vi "SPI Master.vi"(2 "Data In U32":u32, 3 "Data In U64":u64, 4 "Mode":bool) -> (0 "Data In Out U32":u32, 1 "Data In Out U64":u64)   [LabVIEW 2018]
uses:
  <vilib>/rvi/eio/common/nirviEmuTemplateMethod_errors.vi
  <vilib>/eio/EIONode/EIONode.xnode
panel:
  # "ON = 8 Bits SPI\nOFF = 16 Bits SPI"
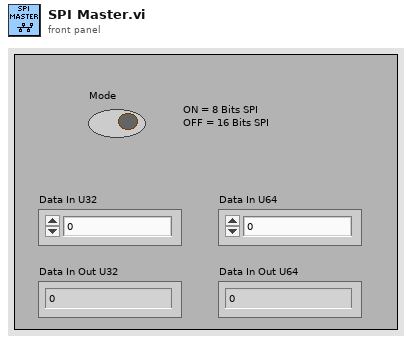
[diagram p1: front panel]
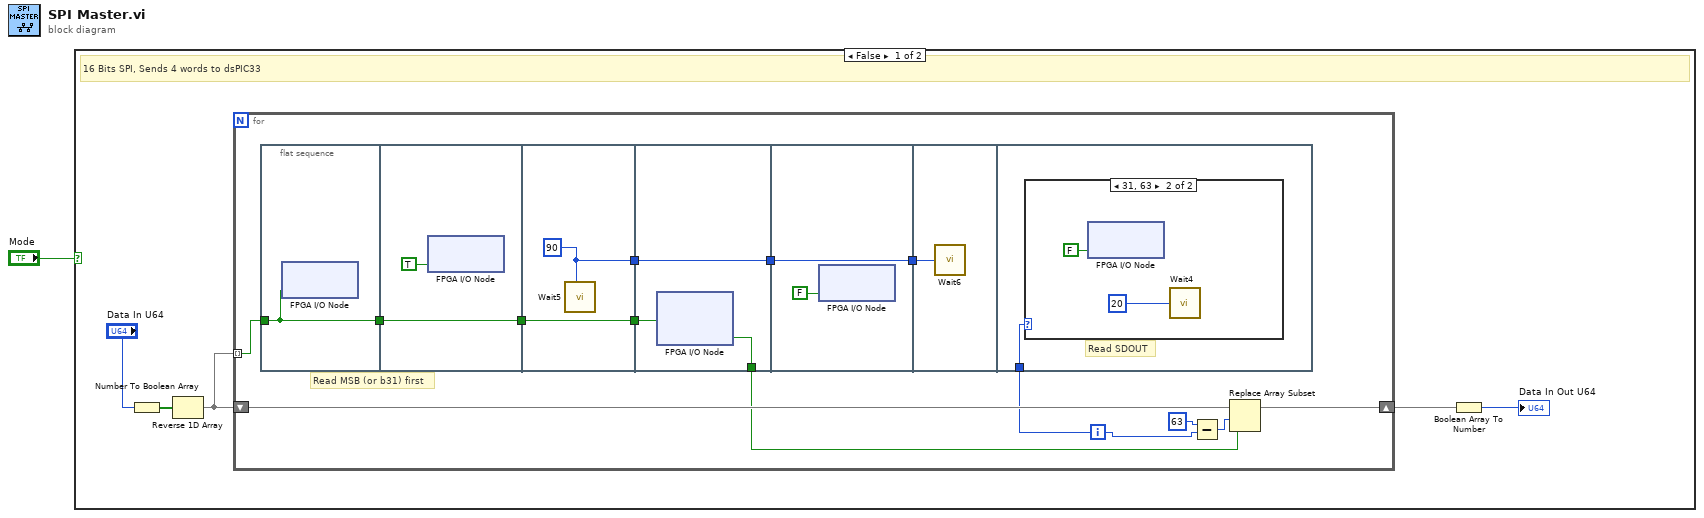
[diagram p0: block diagram]
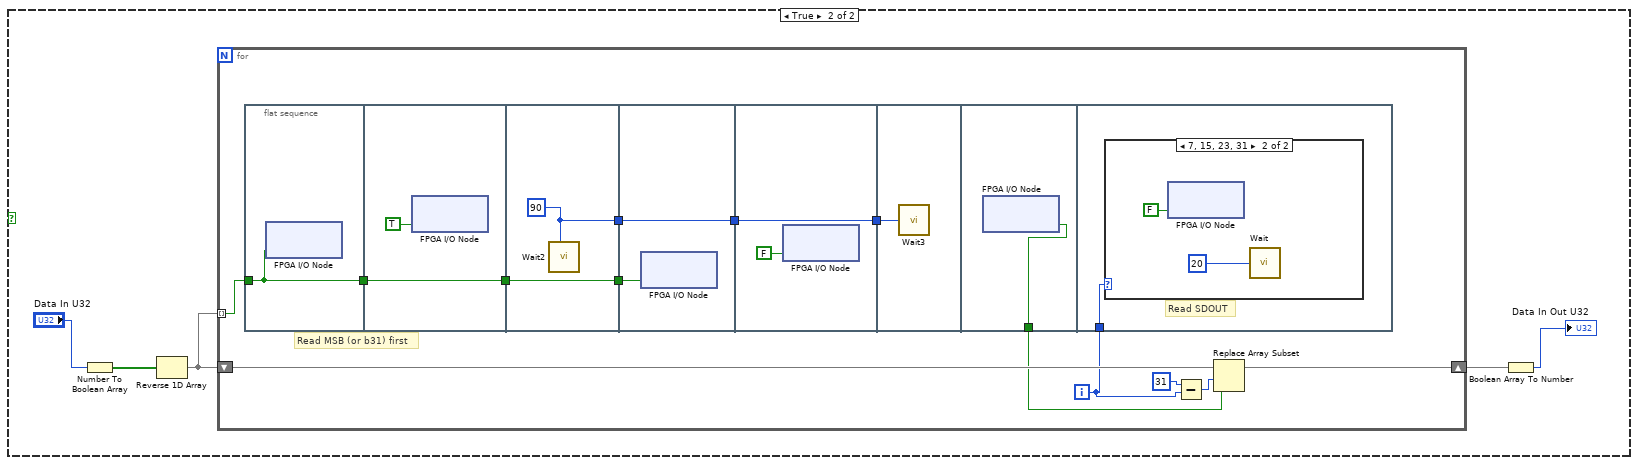
[diagram p3: hidden frame]
diagram:
  n1 = case shown="False" "Mode" {
    frame False {
      # "16 Bits SPI, Sends 4 words to dsPIC33"
      n2 = Number To Boolean Array(number="Data In U64") -> (Boolean array=w4:bool[])
      n3 = Reverse 1D Array(array=w4) -> (reversed array=w5:bool[])
      n4 = for {
        shift-right: [w18] -> w6
        shift-left: w5 -> [w19]
        tunnel: w5 -> [w15] mode=indexing
        i -> [w14]
        # "Read MSB (or b31) first"
        n5 = flat-sequence {
          tunnel: [w20] -> w11
          tunnel: w15 -> [w20]
          tunnel: w11 -> [w22]
          tunnel: [w22] -> w10
          tunnel: w10 -> [w24]
          tunnel: [w24] -> w13
          tunnel: [w23] -> w12
          tunnel: w13 -> [w27]
          tunnel: [w26] -> w9
          tunnel: w12 -> [w26]
          tunnel: [w25] -> w7
          tunnel: w9 -> [w29]
          tunnel: [w29] -> w8
          tunnel: w8 -> [w30]
          tunnel: w14 -> [w31]
          frame #0 {
            n6 = xnode "FPGA I/O Node"("MOSI"=w20) -> ()  [unwired: 1 in, 1 out]
          }
          frame #1 {
            n7 = xnode "FPGA I/O Node"("SCLK"=TRUE) -> ()  [unwired: 1 in, 1 out]
          }
          frame #2 {
            w23 = u8 90 ("Delay")
            n8 = call "Wait5"("Count(Ticks)"=w23) -> ()  [unwired: 1 out]
          }
          frame #3 {
            n9 = xnode "FPGA I/O Node"("MOSI"=w27) -> ("MISO"=w25:bool)  [unwired: 2 in, 2 out]
          }
          frame #4 {
            n10 = xnode "FPGA I/O Node"("SCLK"=FALSE) -> ()  [unwired: 1 in, 1 out]
          }
          frame #5 {
            n11 = call "Wait6"("Count(uSec)"=w30) -> ()  [unwired: 1 out]
          }
          frame #6 {
            # "Read SDOUT"
            n12 = case shown="31, 63" w31 {
              frame 0, Default {
              }
              frame 31, 63 {
                n13 = xnode "FPGA I/O Node"("MOSI"=FALSE) -> ()  [unwired: 1 in, 1 out]
                n14 = call "Wait4"("Count(Ticks)"=u8 20 ("Count(uSec)")) -> ()  [unwired: 1 out]
              }
            }
          }
        }
        n15 = Subtract(x=63, y=w14) -> (x-y=w16:i32)
        n16 = Replace Array Subset(array=w19, new element=w7, index=w16) -> (w18:bool[])
      }
      n17 = Boolean Array To Number(Boolean array=w6) -> (number=→"Data In Out U64":u64)
    }
    frame True {
      n18 = Number To Boolean Array(number="Data In U32") -> (Boolean array=w36:bool[])
      n19 = Reverse 1D Array(array=w36) -> (reversed array=w37:bool[])
      n20 = for {
        shift-right: [w50] -> w38
        shift-left: w37 -> [w51]
        tunnel: w37 -> [w47] mode=indexing
        i -> [w46]
        # "Read MSB (or b31) first"
        n21 = flat-sequence {
          tunnel: [w52] -> w43
          tunnel: w47 -> [w52]
          tunnel: w43 -> [w54]
          tunnel: [w54] -> w42
          tunnel: w42 -> [w56]
          tunnel: [w56] -> w45
          tunnel: [w55] -> w44
          tunnel: w45 -> [w58]
          tunnel: [w57] -> w41
          tunnel: w44 -> [w57]
          tunnel: w41 -> [w60]
          tunnel: [w60] -> w40
          tunnel: w40 -> [w61]
          tunnel: [w62] -> w39
          tunnel: w46 -> [w63]
          frame #0 {
            n22 = xnode "FPGA I/O Node"("MOSI"=w52) -> ()  [unwired: 1 in, 1 out]
          }
          frame #1 {
            n23 = xnode "FPGA I/O Node"("SCLK"=TRUE) -> ()  [unwired: 1 in, 1 out]
          }
          frame #2 {
            w55 = u8 90 ("Delay")
            n24 = call "Wait2"("Count(Ticks)"=w55) -> ()  [unwired: 1 out]
          }
          frame #3 {
            n25 = xnode "FPGA I/O Node"("MOSI"=w58) -> ()  [unwired: 1 in, 1 out]
          }
          frame #4 {
            n26 = xnode "FPGA I/O Node"("SCLK"=FALSE) -> ()  [unwired: 1 in, 1 out]
          }
          frame #5 {
            n27 = call "Wait3"("Count(uSec)"=w61) -> ()  [unwired: 1 out]
          }
          frame #6 {
            n28 = xnode "FPGA I/O Node"() -> ("MISO"=w62:bool)  [unwired: 1 in, 1 out]
          }
          frame #7 {
            # "Read SDOUT"
            n29 = case shown="7, 15, 23, 31" w63 {
              frame 0, Default {
              }
              frame 7, 15, 23, 31 {
                n30 = xnode "FPGA I/O Node"("MOSI"=FALSE) -> ()  [unwired: 1 in, 1 out]
                n31 = call "Wait"("Count(Ticks)"=u8 20 ("Count(uSec)")) -> ()  [unwired: 1 out]
              }
            }
          }
        }
        n32 = Subtract(x=31, y=w46) -> (x-y=w48:i32)
        n33 = Replace Array Subset(array=w51, new element=w39, index=w48) -> (w50:bool[])
      }
      n34 = Boolean Array To Number(Boolean array=w38) -> (number=→"Data In Out U32":u32)
    }
  }
